vi "configuration_manager.vi"(8 "error in (no error)":errorcluster, 11 "user":string(xcontrol)="default") -> (0 "error out":errorcluster)   [LabVIEW 2010]
doc: "Set here the configuration of the HelioScan framework."
uses:
  common/xcontrols/XUserDropdown/XUserDropdown/XUserDropdown.xctl
  controls/button_edit.ctl
  controls/button_rename.ctl
  controls/button_create.ctl
  controls/button_add.ctl
  controls/button_delete.ctl
  controls/button_collapse.ctl
  common/classes/ErrorController/ErrorController/ErrorController.lvclass
  common/clusters/plugin_specification.ctl
  common/classes/GenericComponent/GenericComponent/GenericComponent.lvclass
  common/classes/ErrorController/ErrorController/class_data.vi
  kernel32.dll
panel:
  in  "button:collapse_all":T1
  in  "button:rename":T2
  in  "button: create new item":T3
  in  "button: add item":T4
  in  "button: copy user":bool
  in  "button: delete user":bool
  in  "button: new user":bool
  in  "button: edit component configuration":T5
  in  "button: delete component configuration":T6
  in  "component configurations":string(tree) caption="Existing configurations"
  in  "button: edit top-level configuration":bool
  out "error loaded?":bool
  in  "done button":bool
  out "loading progress bar":u8(slide) scale=0.0..100.0
  # "Configuration Manager"
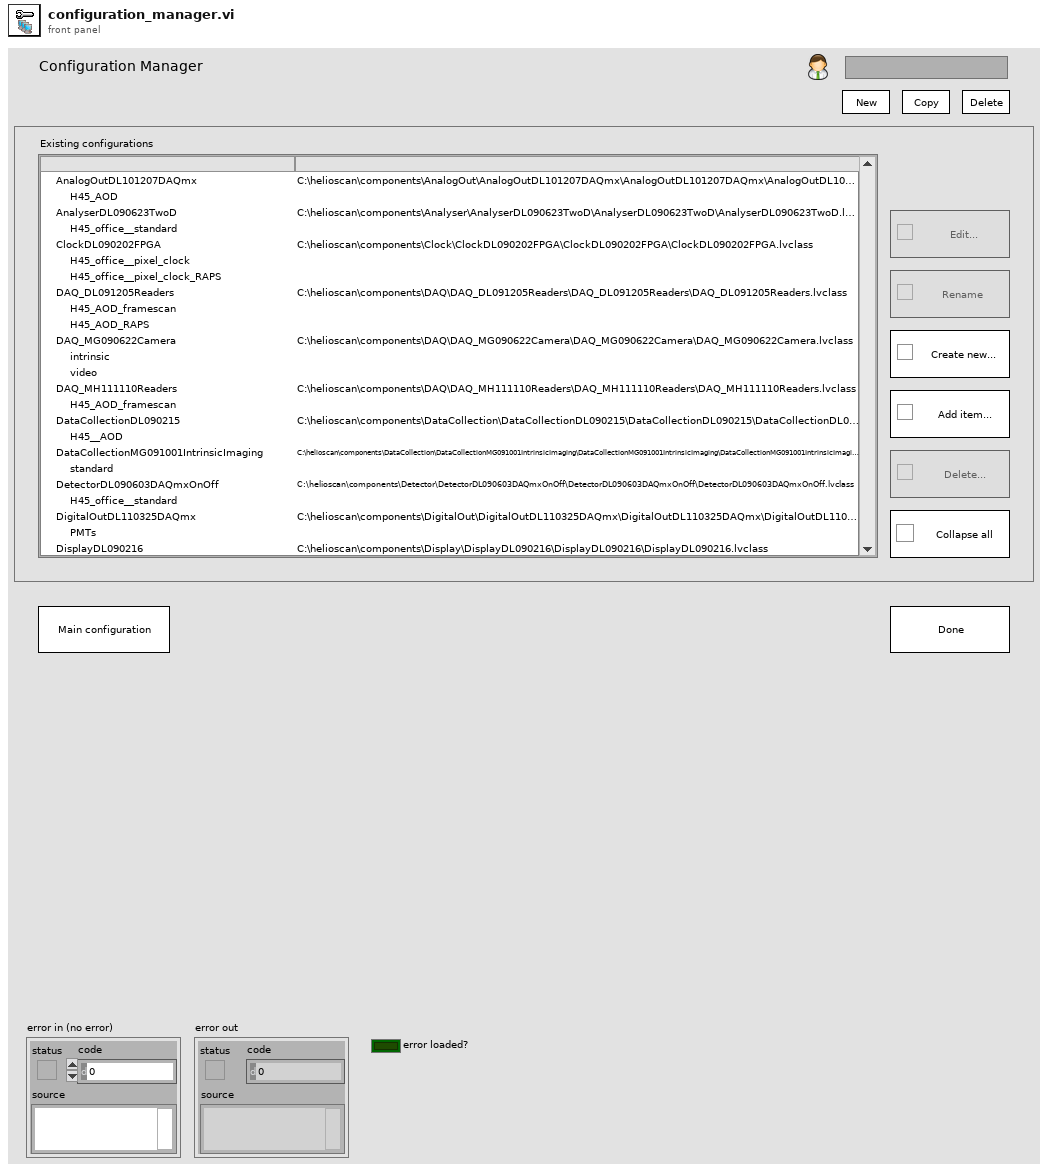
[diagram p1: front panel]
types:
  T1 = typedef "button_collapse.ctl" = bool
  T2 = typedef "button_rename.ctl" = bool
  T3 = typedef "button_create.ctl" = bool
  T4 = typedef "button_add.ctl" = bool
  T5 = typedef "button_edit.ctl" = bool
  T6 = typedef "button_delete.ctl" = bool
  T7 = enum8{"Enabled", "Disabled", "Disabled and Grayed Out"}
  T8 = typedef "plugin_specification.ctl" = cluster{"class path":string, "configuration":string, "label":string, "settings name":string}
  T9 = typedef "configuration_paths_cluster.ctl" = cluster{"base folder":path, "base folder for user":path, "component folder":path, "component file path":path, "main folder":path, "main file":path}
  T10 = typedef "component_path_clusters.ctl" = cluster{"components directory":path, "component type directory":path, "specific component directory":path, "component class path":path}
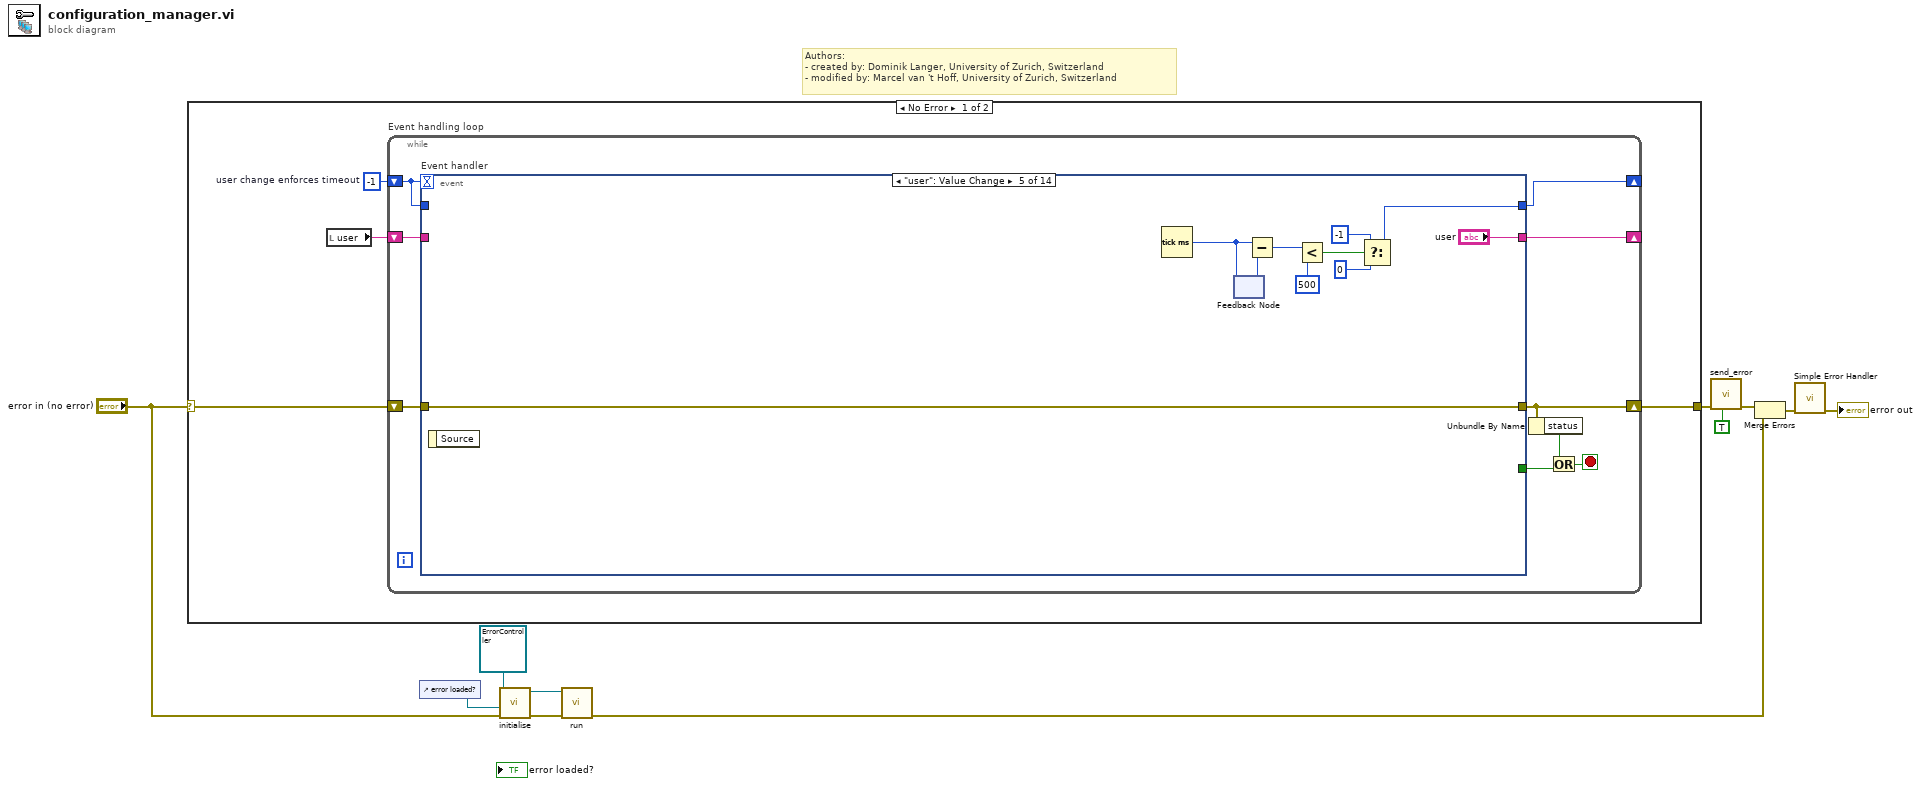
[diagram p0: block diagram]
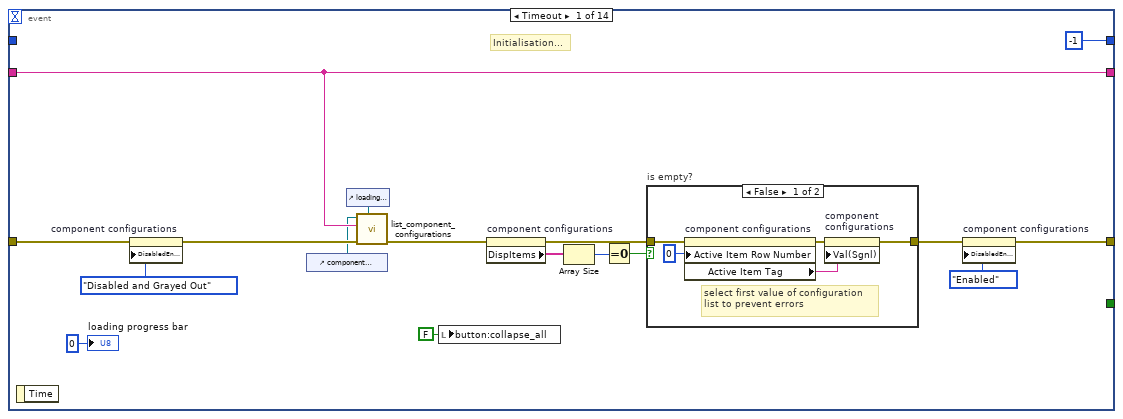
[diagram p2: hidden frame]
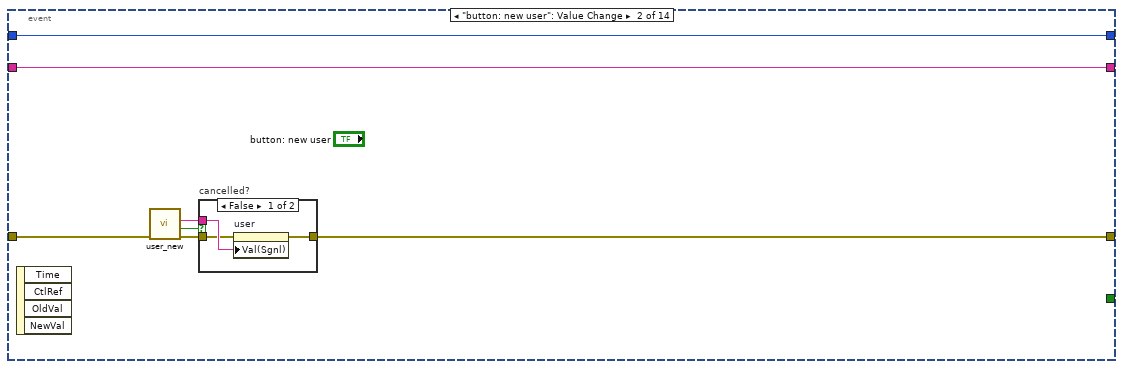
[diagram p4: hidden frame]
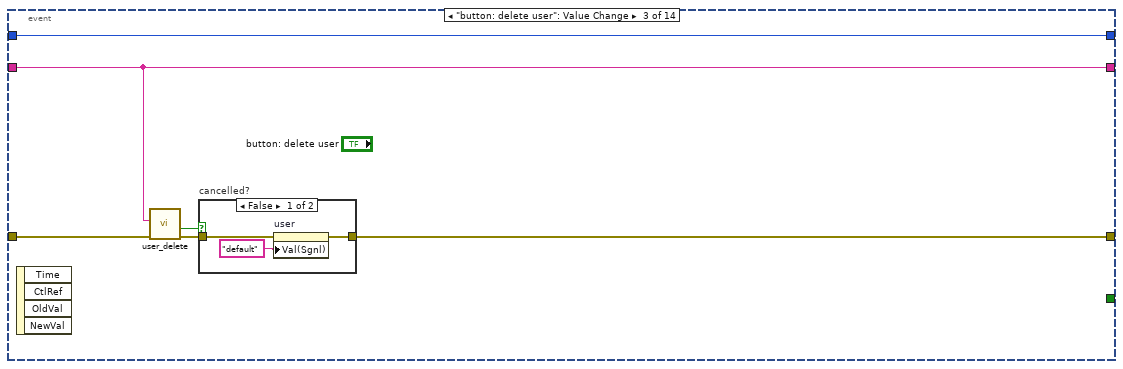
[diagram p6: hidden frame]
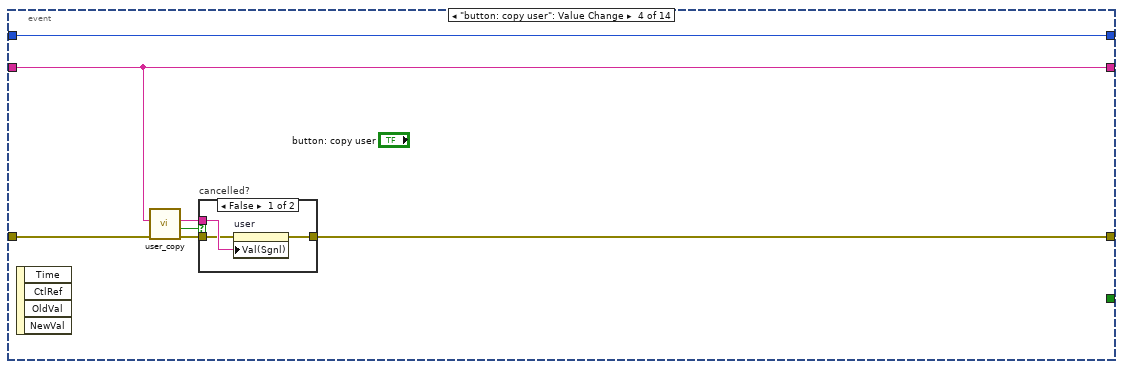
[diagram p8: hidden frame]
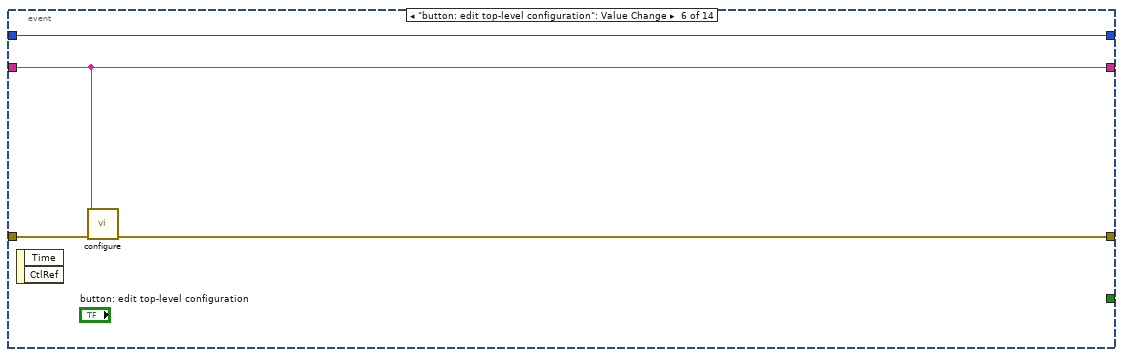
[diagram p10: hidden frame]
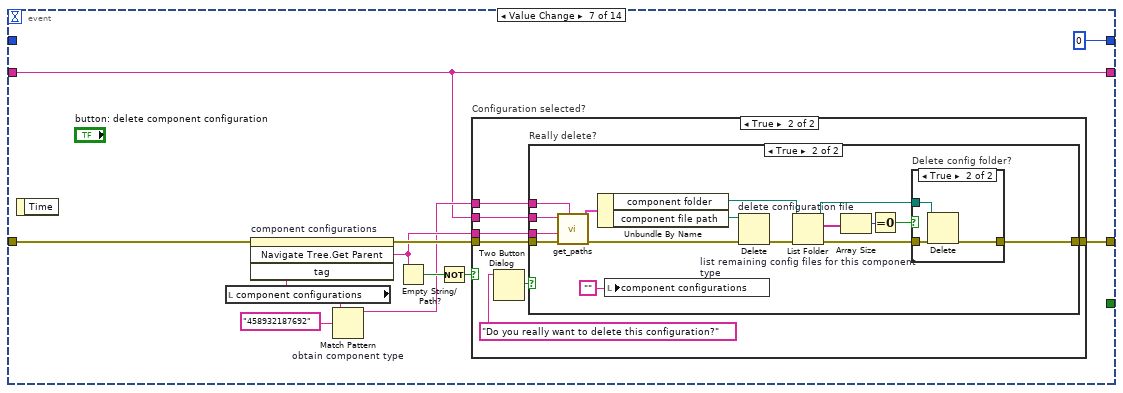
[diagram p11: hidden frame]
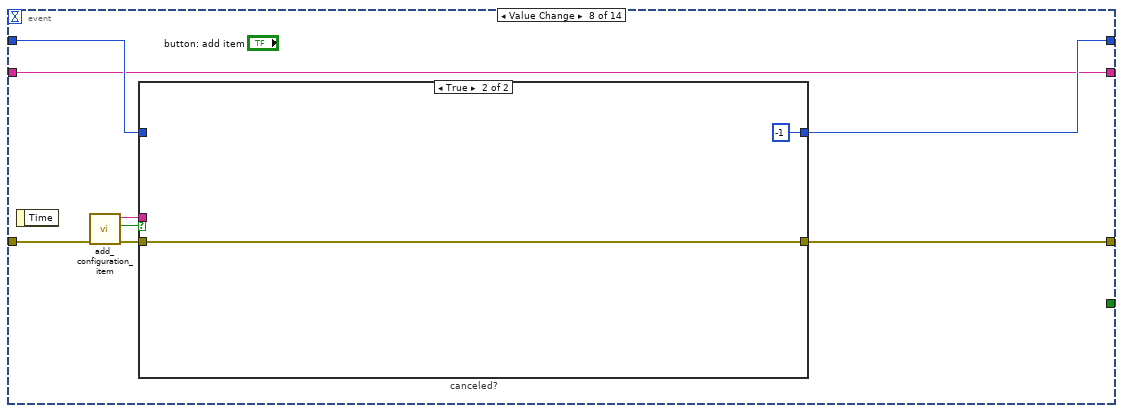
[diagram p15: hidden frame]
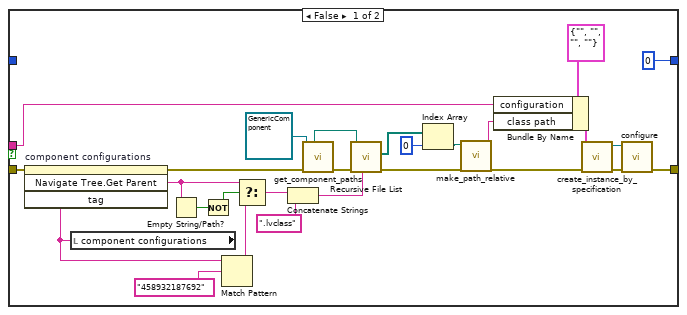
[diagram p16: hidden frame]
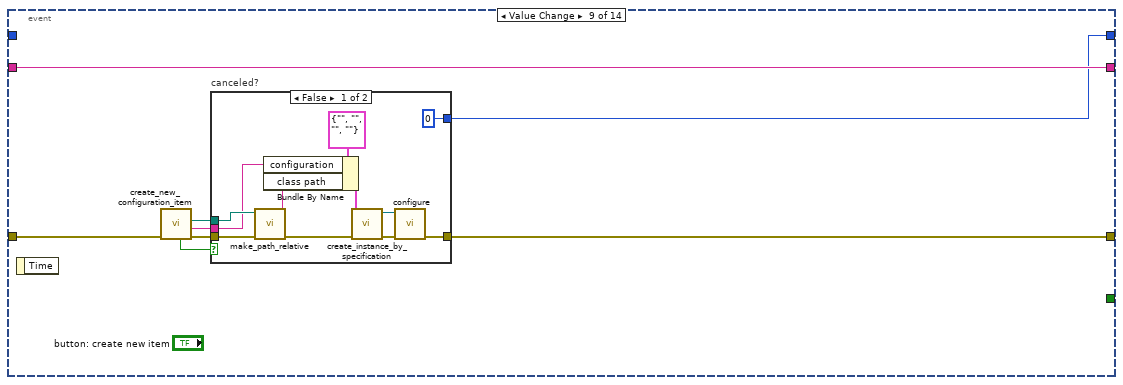
[diagram p17: hidden frame]
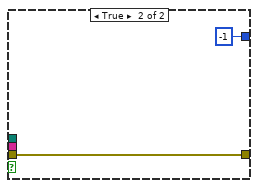
[diagram p18: hidden frame]
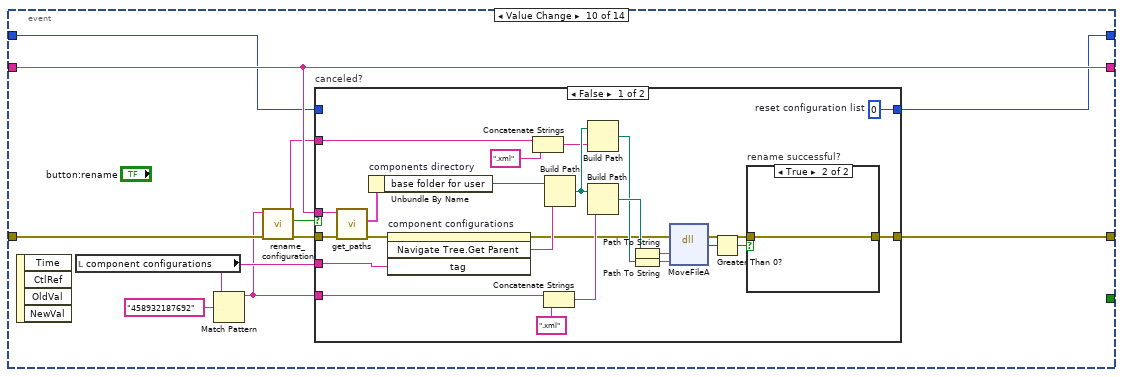
[diagram p19: hidden frame]
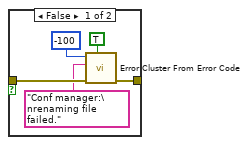
[diagram p20: hidden frame]
diagram:
  # "Authors: \n- created by: Dominik Langer, University of Zurich, Switzerland\n- modified by: Marcel van 't Hoff, University of Zurich, Switzerland"
  n1 = case shown="No Error" "error in (no error)" {
    selector: "error in (no error)" -> [w14 w307]
    tunnel: [w13 w307] -> w10
    frame No Error {
      w15 = -1  # user change enforces timeout
      n2 = local read "user"() -> (w12:string)
      n3 = while "Event handling loop" {
        shift-right: [w23] -> _
        shift-left: w15 -> [w17]
        shift-right: [w19] -> _
        shift-left: w12 -> [w18]
        shift-right: [w16] -> w13
        shift-left: w14 -> [w24]
        stop <- w21 stop-if-true
        n4 = event "Event handler" shown="[4] \"user\": Value Change" {
          selector: _ -> [_ _ _ _ _ _ _ _ _ _ _ _ _ _]
          dyn-events: _ -> [_ _ _ _ _ _ _ _ _ _ _ _ _ _]
          timeout: w17 -> [_ _ _ _ _ _ _ _ _ _ _ _ _ _]
          tunnel: w24 -> [w38 w52 w63 w74 w88 w92 w103 w137 w177 w202 w240 w272 w299 w304]
          tunnel: [-1 w54 w64 w75 w80 w93 0 w140 w171 w194 w241 w273 w300 w306] -> w23
          tunnel: w17 -> [_ w54 w64 w75 _ w93 _ w139 _ w193 w241 w273 w300 w306]
          tunnel: [w35 w48 w60 w71 w88 w91 w100 w141 w173 w199 w239 w270 w299 w303] -> w16
          tunnel: [_ _ _ _ _ _ _ _ _ _ _ _ TRUE _] -> w20
          tunnel: [w40 w53 w62 w70 "user" w90 w95 w138 w178 w200 w235 w265 w297 w305] -> w19
          tunnel: w18 -> [w40 w53 w62 w70 _ w90 w95 w138 w178 w200 w235 w265 w297 w305]
          event Timeout {
            # "Initialisation..."
            n5 = event-data() -> ()  [unwired: 2 out]
            n6 = property on="component configurations" class="Tree (strict)"(error in=w38, "DisabledEnum"=T7."Disabled and Grayed Out" ("Disabled")) -> (error out=w33:errorcluster)  [unwired: 1 in, 1 out]
            n7 = control-ref of="component configurations"() -> (w27:refnum<vi>)
            n8 = control-ref of="loading progress bar"() -> (w26:refnum<vi>)
            n9 = call "list_component_configurations.vi"("progress bar ref"=w26, "error in (no error)"=w33, "user name"=w40, "tree ref"=w27) -> ("error out"=w28:errorcluster)  [unwired: 1 in, 6 out]
            n10 = local write "button:collapse_all"(T1 FALSE ("button:collapse_all")) -> ()
            n11 = property on="component configurations" class="Tree (strict)"(error in=w28) -> (error out=w29:errorcluster, "DispItems"=w32:string[])  [unwired: 1 in, 1 out]
            n12 = Array Size(array=w32) -> (size(s)=w31:i32)
            n13 = Equal To 0?(x=w31) -> (x = 0?=w30:bool)
            n14 = case "is empty?" shown="False" w30 {
              tunnel: [w46 w47] -> w36
              tunnel: w29 -> [w44 w47]
              frame False {
                # "select first value of configuration\nlist to prevent errors"
                n15 = property on="component configurations" class="Tree (strict)"(error in=w44, "Active Item Row Number"=0 ("Active Item:Row Number")) -> (error out=w43:errorcluster, "Active Item Tag"=w42:string)  [unwired: 1 in, 1 out]
                n16 = property on="component \nconfigurations" class="Tree (strict)"(error in=w43, "Val(Sgnl)"=w42) -> (error out=w46:errorcluster)  [unwired: 1 in, 1 out]
              }
              frame True {
              }
            }
            n17 = property on="component configurations" class="Tree (strict)"(error in=w36, "DisabledEnum"=T7."Enabled" ("Disabled")) -> (error out=w35:errorcluster)  [unwired: 1 in, 1 out]
            "loading progress bar" <- u8 0 ("loading progress bar")
          }
          event "button: new user": Value Change {
            n18 = event-data() -> ()  [unwired: 5 out]
            n19 = call "user_new.vi"("error in (no error)"=w52) -> ("error IO"=w49:errorcluster, "cancelled?"=w51:bool, "user name out"=w50:string)  [unwired: 8 in]
            n20 = case "cancelled?" shown="False" w51 {
              tunnel: w50 -> [w57 _]
              tunnel: w49 -> [w56 w58]
              tunnel: [w55 w58] -> w48
              frame False {
                n21 = property on="user" class="XUserDropdown (strict)"(error in=w56, "Val(Sgnl)"=w57) -> (error out=w55:errorcluster)  [unwired: 1 in, 1 out]
              }
              frame True {
              }
            }
          }
          event "button: delete user": Value Change {
            n22 = event-data() -> ()  [unwired: 5 out]
            n23 = call "user_delete.vi"("error in (no error)"=w63, "user name in"=w62) -> ("error out"=w61:errorcluster, "cancelled?"=w59:bool)  [unwired: 8 in]
            n24 = case "cancelled?" shown="False" w59 {
              tunnel: w61 -> [w67 w68]
              tunnel: [w66 w68] -> w60
              frame False {
                n25 = property on="user" class="XUserDropdown (strict)"(error in=w67, "Val(Sgnl)"="default" ("Value (Signaling)")) -> (error out=w66:errorcluster)  [unwired: 1 in, 1 out]
              }
              frame True {
              }
            }
          }
          event "button: copy user": Value Change {
            n26 = event-data() -> ()  [unwired: 5 out]
            n27 = call "user_copy.vi"("error in (no error)"=w74, "old user name in"=w70) -> ("error out"=w73:errorcluster, "cancelled?"=w69:bool, "new user name out"=w72:string)  [unwired: 7 in]
            n28 = case "cancelled?" shown="False" w69 {
              tunnel: w72 -> [w78 _]
              tunnel: w73 -> [w77 w79]
              tunnel: [w76 w79] -> w71
              frame False {
                n29 = property on="user" class="XUserDropdown (strict)"(error in=w77, "Val(Sgnl)"=w78) -> (error out=w76:errorcluster)  [unwired: 1 in, 1 out]
              }
              frame True {
              }
            }
          }
          event "user": Value Change {
            n30 = event-data() -> ()  [unwired: 2 out]
            n31 = Tick Count (ms)() -> (millisecond timer value=w87:u32)
            n32 = feedback-in #1(w87) -> ()
            n33 = feedback #1() -> (w86:u32)  [unwired: 1 in]
            n34 = Subtract(x=w87, y=w86) -> (x-y=w85:u32)
            n35 = Less?(x=w85, y=u32 500) -> (x < y?=w83:bool)
            n36 = Select(t=-1 ("reset configuration list"), s=w83, f=0) -> (s? t:f=w80:i32)
          }
          event "button: edit top-level configuration": Value Change {
            n37 = event-data() -> ()  [unwired: 3 out]
            n38 = call "configure.vi"("error in (no error)"=w92, "user"=w90) -> ("error out"=w91:errorcluster)  [unwired: 1 in, 8 out]
          }
          event Value Change {
            n39 = event-data() -> ()  [unwired: 2 out]
            n40 = local read "component configurations"() -> (w98:string)
            n41 = invoke on="component configurations" class="Tree (strict)" method="Navigate Tree.Get Parent"(error in=w103, "tag"=w98) -> (error out=w102:errorcluster, "Navigate Tree:Get Parent"=w99:string)  [unwired: 2 in, 2 out]
            n42 = Match Pattern "obtain component type"(string=w98, regular expression="458932187692") -> (before substring=w97:string)  [unwired: 4 out]
            n43 = Empty String/Path?(string/path=w99) -> (empty?=w104:bool)
            n44 = Not(x=w104) -> (.not. x?=w101:bool)
            n45 = case "Configuration selected?" shown="True" w101 {
              tunnel: w102 -> [w105 w112]
              tunnel: w97 -> [_ w110]
              tunnel: [w105 w109] -> w100
              tunnel: w99 -> [_ w111]
              tunnel: w95 -> [_ w106]
              frame False {
              }
              frame True {
                n46 = Two Button Dialog(message="Do you really want to delete this configuration?") -> (T button?=w108:bool)  [unwired: 2 out]
                n47 = case "Really delete?" shown="True" w108 {
                  tunnel: w112 -> [w113 w128]
                  tunnel: w111 -> [_ w120]
                  tunnel: w110 -> [_ w115]
                  tunnel: [w113 w123] -> w109
                  tunnel: w106 -> [_ w116]
                  frame False {
                  }
                  frame True {
                    n48 = call "get_paths.vi"("configuration file name (without ending)"=w115, "error in (no error)"=w128, "component name"=w120, "user"=w116) -> ("error out"=w129:errorcluster, "configuration paths"=w119:T9)  [unwired: 4 in, 2 out]
                    n49 = Unbundle By Name(w119) -> ("component folder"=w117:path, "component file path"=w118:path)
                    n50 = local write "component configurations"("") -> ()
                    n51 = Delete "delete configuration file"(path (use dialog)=w118, error in=w129) -> (error out=w127:errorcluster)  [unwired: 5 out]
                    n52 = List Folder "list remaining config files for this component type"(path=w117, error in=w127) -> (path out=w121:path, filenames=w126:string[], error out=w124:errorcluster)  [unwired: 3 out]
                    n53 = Array Size(array=w126) -> (size(s)=w125:i32)
                    n54 = Equal To 0?(x=w125) -> (x = 0?=w122:bool)
                    n55 = case "Delete config folder?" shown="True" w122 {
                      tunnel: w124 -> [w130 w133]
                      tunnel: [w130 w132] -> w123
                      tunnel: w121 -> [_ w131]
                      frame False {
                      }
                      frame True {
                        n56 = Delete(path (use dialog)=w131, error in=w133) -> (error out=w132:errorcluster)  [unwired: 5 out]
                      }
                    }
                  }
                }
              }
            }
          }
          event Value Change {
            n57 = event-data() -> ()  [unwired: 2 out]
            n58 = call "add_configuration_item.vi"("error in (no error)"=w137) -> ("error out"=w136:errorcluster, "canceled?"=w134:bool, "additional-component config name 2"=w135:string)  [unwired: 8 in]
            n59 = case "canceled?" shown="True" w134 {
              tunnel: [w167 w170] -> w141
              tunnel: [0 -1] -> w140
              tunnel: w139 -> [_ _]
              tunnel: w136 -> [w163 w170]
              tunnel: w135 -> [w142 _]
              frame False {
                n60 = local read "component configurations"() -> (w165:string)
                n61 = invoke on="component configurations" class="Tree (strict)" method="Navigate Tree.Get Parent"(error in=w163, "tag"=w165) -> (error out=w168:errorcluster, "Navigate Tree:Get Parent"=w158:string)  [unwired: 2 in, 2 out]
                n62 = Empty String/Path?(string/path=w158) -> (empty?=w162:bool)
                n63 = Not(x=w162) -> (.not. x?=w160:bool)
                n64 = Match Pattern(string=w165, regular expression="458932187692") -> (before substring=w159:string)  [unwired: 4 out]
                n65 = Select(t=w158, s=w160, f=w159) -> (s? t:f=w161:string)
                n66 = Concatenate Strings(w161, ".lvclass" ("string")) -> (w156:string)
                n67 = call-dynamic "get_component_paths.vi"("error in (no error)"=w168, "GenericComponent in"=refnum<class "GenericComponent.lvclass"> refnum ("GenericComponent.lvclass")) -> ("error out"=w153:errorcluster, "components directory"=w152:path)  [unwired: 4 in, 4 out]
                n68 = call <vilib>:"Recursive File List.vi"("pattern"=w156, "error in (no error)"=w153, "Folder Path"=w152) -> ("error out"=w146:errorcluster, "All Files in Dir"=w155:path[])  [unwired: 1 in, 6 out]
                n69 = Index Array(array=w155, index=0) -> (element=w144:path)
                n70 = call "make_path_relative.vi"("error in (no error)"=w146, "absolute path"=w144) -> ("error out"=w145:errorcluster, "relative path"=w143:string)  [unwired: 8 in]
                n71 = Bundle By Name(cluster=T8 {"class path"="", "configuration"="", "label"="", "settings name"=""} ("component specification"), "configuration"=w142, "class path"=w143) -> (w150:T8)
                n72 = call "create_instance_by_specification.vi"("error in (no error)"=w145, "component specification"=w150) -> ("error out"=w148:errorcluster, "GenericPlugin out"=w147:refnum<class "GenericComponent.lvclass">)  [unwired: 7 in, 1 out]
                n73 = call-dynamic "configure.vi"("error in (no error)"=w148, "GenericPlugin in"=w147) -> ("error out"=w167:errorcluster)  [unwired: 9 out]
              }
              frame True {
              }
            }
          }
          event Value Change {
            n74 = event-data() -> ()  [unwired: 2 out]
            n75 = call "create_new_configuration_item.vi"("error in (no error)"=w177) -> ("error out"=w176:errorcluster, "new-component config name out"=w174:string, "component path out"=w175:path, "canceled?"=w172:bool)  [unwired: 7 in]
            n76 = case "canceled?" shown="False" w172 {
              tunnel: w176 -> [w184 w191]
              tunnel: w175 -> [w183 _]
              tunnel: w174 -> [w182 _]
              tunnel: [w180 w191] -> w173
              tunnel: [0 -1] -> w171
              frame False {
                n77 = call "make_path_relative.vi"("error in (no error)"=w184, "absolute path"=w183) -> ("error out"=w187:errorcluster, "relative path"=w181:string)  [unwired: 8 in]
                n78 = Bundle By Name(cluster=T8 {"class path"="", "configuration"="", "label"="", "settings name"=""} ("component specification"), "configuration"=w182, "class path"=w181) -> (w188:T8)
                n79 = call "create_instance_by_specification.vi"("error in (no error)"=w187, "component specification"=w188) -> ("error out"=w186:errorcluster, "GenericPlugin out"=w185:refnum<class "GenericComponent.lvclass">)  [unwired: 7 in, 1 out]
                n80 = call-dynamic "configure.vi"("error in (no error)"=w186, "GenericPlugin in"=w185) -> ("error out"=w180:errorcluster)  [unwired: 9 out]
              }
              frame True {
              }
            }
          }
          event Value Change {
            n81 = event-data() -> ()  [unwired: 5 out]
            n82 = local read "component configurations"() -> (w196:string)
            n83 = Match Pattern(string=w196, regular expression="458932187692") -> (before substring=w195:string)  [unwired: 4 out]
            n84 = call "rename_configuration.vi"("error in (no error)"=w202, "old name in"=w195) -> ("error out"=w201:errorcluster, "canceled?"=w198:bool, "new name out"=w197:string)  [unwired: 7 in]
            n85 = case "canceled?" shown="False" w198 {
              tunnel: w201 -> [w206 w234]
              tunnel: w196 -> [w222 _]
              tunnel: w200 -> [w226 _]
              tunnel: [w205 w234] -> w199
              tunnel: w197 -> [w213 _]
              tunnel: w195 -> [w220 _]
              tunnel: [w204 w233] -> w194
              tunnel: w193 -> [_ w233]
              frame False {
                w204 = 0  # reset configuration list
                n86 = call "get_paths.vi"("error in (no error)"=w206, "user"=w226) -> ("error out"=w207:errorcluster, "configuration paths"=w225:T9)  [unwired: 6 in, 2 out]
                n87 = Unbundle By Name "components directory"(w225) -> ("base folder for user"=w224:path)
                n88 = invoke on="component configurations" class="Tree (strict)" method="Navigate Tree.Get Parent"(error in=w207, "tag"=w222) -> (error out=w203:errorcluster, "Navigate Tree:Get Parent"=w223:string)  [unwired: 2 in, 2 out]
                n89 = Concatenate Strings(w213, ".xml" ("string")) -> (w212:string)
                n90 = Concatenate Strings(w220, ".xml" ("string")) -> (w219:string)
                n91 = Build Path(base path=w224, name or relative path=w223) -> (appended path=w215:path)
                n92 = Build Path(base path=w215, name or relative path=w212) -> (appended path=w211:path)
                n93 = Build Path(base path=w215, name or relative path=w219) -> (appended path=w216:path)
                n94 = Path To String(path=w216) -> (string=w218:string)
                n95 = Path To String(path=w211) -> (string=w217:string)
                n96 = dll-call lib="kernel32.dll" fn="MoveFileA" label="rename file"(error in=w203, w218, w217) -> (error out=w209:errorcluster, w210:i32)  [unwired: 4 in, 1 out]
                n97 = Greater Than 0?(x=w210) -> (x > 0?=w208:bool)
                n98 = case "rename successful?" shown="True" w208 {
                  tunnel: w209 -> [w231 w232]
                  tunnel: [w230 w232] -> w205
                  frame False {
                    n99 = call <vilib>:"Error Cluster From Error Code.vi"("show call chain? (False)"=TRUE, "error in (no error)"=w231, "error message (\"\")"="Conf manager:\nrenaming file failed." ("error message (\"\")"), "error code (0)"=-100) -> ("error out"=w230:errorcluster)  [unwired: 5 in]
                  }
                  frame True {
                  }
                }
              }
              frame True {
              }
            }
          }
          event "component configurations": Value Change {
            n100 = event-data() -> ()  [unwired: 2 out]
            n101 = Empty String/Path?(string/path="component configurations") -> (empty?=w237:bool)
            n102 = Not(x=w237) -> (.not. x?=w236:bool)
            n103 = case "Valid node selected?" shown="True" w236 {
              tunnel: w240 -> [w244 w263]
              tunnel: [w243 w254] -> w239
              tunnel: "component configurations" -> [_ w259]
              frame False {
                n104 = control-ref of="button: add item"() -> (w247:refnum<vi>)
                n105 = call "bool_to_enable_state.vi"("boolean in"=FALSE) -> ("enabled status out"=w246:T7)  [unwired: 4 in]
                n106 = Build Array(w247) -> (w242:refnum<vi>[])
                n107 = call "set_disabled_state.vi"("error in"=w244, "status in"=w246, "control references"=w242) -> ("error out"=w243:errorcluster)  [unwired: 8 out]
              }
              frame True {
                n108 = invoke on="component configurations" class="Tree (strict)" method="Navigate Tree.Get Parent"(error in=w263, "tag"=w259) -> (error out=w262:errorcluster, "Navigate Tree:Get Parent"=w264:string)  [unwired: 2 in, 2 out]
                n109 = Empty String/Path?(string/path=w264) -> (empty?=w251:bool)
                n110 = control-ref of="button:rename"() -> (w249:refnum<vi>)
                n111 = control-ref of="button: delete component configuration"() -> (w261:refnum<vi>)
                n112 = control-ref of="button: edit component configuration"() -> (w258:refnum<vi>)
                n113 = Not(x=w251) -> (.not. x?=w252:bool)
                n114 = call "bool_to_enable_state.vi"("boolean in"=w252) -> ("enabled status out"=w250:T7)  [unwired: 4 in]
                n115 = Build Array(w249, w261, w258) -> (w260:refnum<vi>[])
                n116 = call "set_disabled_state.vi"("error in"=w262, "status in"=w250, "control references"=w260) -> ("error out"=w257:errorcluster)  [unwired: 8 out]
                n117 = control-ref of="button: add item"() -> (w256:refnum<vi>)
                n118 = call "bool_to_enable_state.vi"("boolean in"=TRUE) -> ("enabled status out"=w253:T7)  [unwired: 4 in]
                n119 = Build Array(w256) -> (w255:refnum<vi>[])
                n120 = call "set_disabled_state.vi"("error in"=w257, "status in"=w253, "control references"=w255) -> ("error out"=w254:errorcluster)  [unwired: 8 out]
              }
            }
          }
          event "component configurations": Double Click; Value Change {
            n121 = event-data() -> ()  [unwired: 2 out]
            n122 = local read "component configurations"() -> (w269:string)
            n123 = invoke on="component configurations" class="Tree (strict)" method="Navigate Tree.Get Parent"(error in=w272, "tag"=w269) -> (error out=w271:errorcluster, "Navigate Tree:Get Parent"=w268:string)  [unwired: 2 in, 2 out]
            n124 = Empty String/Path?(string/path=w268) -> (empty?=w267:bool)
            n125 = Not(x=w267) -> (.not. x?=w266:bool)
            n126 = case "Configuration selected?" shown="True" w266 {
              tunnel: w271 -> [w274 w280]
              tunnel: [w274 w294] -> w270
              tunnel: w269 -> [_ w292]
              tunnel: w268 -> [_ w293]
              tunnel: w265 -> [_ w277]
              frame False {
              }
              frame True {
                n127 = call "get_paths.vi"("error in (no error)"=w280, "user"=w277) -> ("error out"=w281:errorcluster, "component paths"=w279:T10)  [unwired: 6 in, 2 out]
                n128 = Unbundle By Name "components directory"(w279) -> ("components directory"=w278:path)
                n129 = Concatenate Strings(w293, ".lvclass" ("string")) -> (w290:string)
                n130 = call <vilib>:"Recursive File List.vi"("pattern"=w290, "error in (no error)"=w281, "Folder Path"=w278) -> ("error out"=w285:errorcluster, "All Files in Dir"=w289:path[])  [unwired: 1 in, 6 out]
                n131 = Index Array(array=w289, index=0) -> (element=w283:path)
                n132 = call "make_path_relative.vi"("error in (no error)"=w285, "absolute path"=w283) -> ("error out"=w284:errorcluster, "relative path"=w282:string)  [unwired: 8 in]
                n133 = Match Pattern(string=w292, regular expression="458932187692") -> (before substring=w286:string)  [unwired: 4 out]
                n134 = Bundle By Name(cluster=T8 {"class path"="", "configuration"="", "label"="", "settings name"=""} ("component specification"), "class path"=w282, "configuration"=w286) -> (w288:T8)
                n135 = call "create_instance_by_specification.vi"("error in (no error)"=w284, "component specification"=w288) -> ("error out"=w276:errorcluster, "GenericPlugin out"=w275:refnum<class "GenericComponent.lvclass">)  [unwired: 7 in, 1 out]
                n136 = call-dynamic "configure.vi"("error in (no error)"=w276, "GenericPlugin in"=w275) -> ("error out"=w294:errorcluster)  [unwired: 9 out]
              }
            }
          }
          event "done button": Value Change; Panel Close {
            n137 = event-data() -> ()  [unwired: 2 out]
          }
          event Value Change {
            n138 = event-data() -> ()  [unwired: 7 out]
            n139 = Not(x="button:collapse_all") -> (.not. x?=w301:T1)
            n140 = invoke on="component configurations" class="Tree (strict)" method="Open/Close.Open/Close All"(error in=w304, "Open"=w301) -> (error out=w303:errorcluster)  [unwired: 2 in, 3 out]
          }
        }
        n141 = Unbundle By Name(w16) -> ("status"=w22:bool)
        n142 = Or(x=w22, y=w20) -> (x .or. y?=w21:bool)
      }
    }
    frame Error {
    }
  }
  n143 = control-ref of="error loaded?"() -> (w3:refnum<vi>)
  n144 = call-dynamic "initialise.vi"("error in (no error)"="error in (no error)", "error boolean"=w3, "ErrorController in"=refnum<class "ErrorController.lvclass"> refnum ("ErrorController.lvclass")) -> ("error out"=w1:errorcluster, "ErrorController out"=w2:refnum<class "ErrorController.lvclass">)  [unwired: 7 in]
  n145 = call "run.vi"("error in (no error)"=w1, "ErrorController in"=w2) -> ("error out"=w8:errorcluster)  [unwired: 8 in, 1 out]
  n146 = call "send_error.vi"("last error? (F)"=TRUE, "error in (no error)"=w10) -> ("error out"=w9:errorcluster)  [unwired: 9 in]
  n147 = Merge Errors(w9, w8) -> (w6:errorcluster)
  n148 = call <vilib>:"Simple Error Handler.vi"("error in (no error)"=w6) -> ("error out"=→"error out":errorcluster)  [unwired: 4 in, 4 out]
